vi "TCP-IP Mgr.Send.vi"(8 "error in":errorcluster, 10 "Send Data":string) -> (0 "error out":errorcluster)   [LabVIEW 2017, in "TCP-IP Mgr.lvlib"]
uses:
  TCP-IP Mgr.lvlib
  <vilib>/KATE/Queues/Queue Utils.lvlib
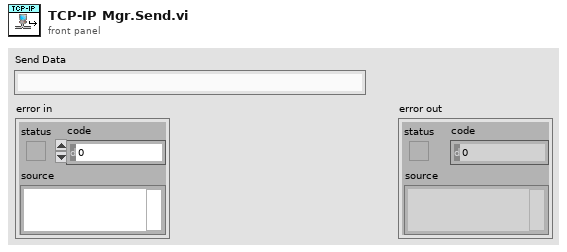
[diagram p1: front panel]
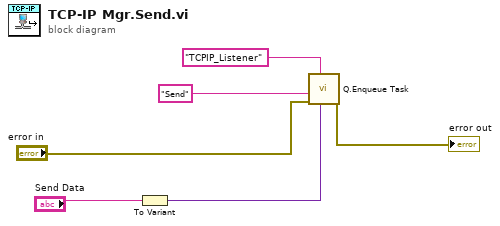
[diagram p0: block diagram]
diagram:
  n1 = To Variant(anything="Send Data") -> (Variant=w3:variant)
  n2 = call <vilib>:"Q.Enqueue Task.vi"("Data1"=w3, "Q Name"="TCPIP_Listener" ("name (unnamed)"), "Error In"="error in", "Task Name"="Send") -> ("error out"=→"error out":errorcluster)  [unwired: 6 in, 1 out]
